vi "Construct.vi"(8 "error in":errorcluster, 11 "board properties in":T1 {"portConfig" items=["FDX_SINGLE", "FDX_REDUNDANT"]; "portSpeed" items=["FDX_100MBIT", "FDX_10MBIT", "FDX_AUTO_100MBIT", "FDX_AUTO_10MBIT", "FDX_AUTO_ERROR", "FDX_1000MBIT"]}) -> (0 "error out":errorcluster, 3 "Shared Resources out":refnum<class "Shared Resources.lvclass">)   [LabVIEW 2020, in "AIM ARINC 664 Engine.lvlib" / "Implementation.lvlib" / "Shared Resources.lvclass"]
uses:
  Shared Resources.lvclass
  Import/_typedefs/board_setup.ctl
  Import/AIM ARINC 664 Import.lvlib
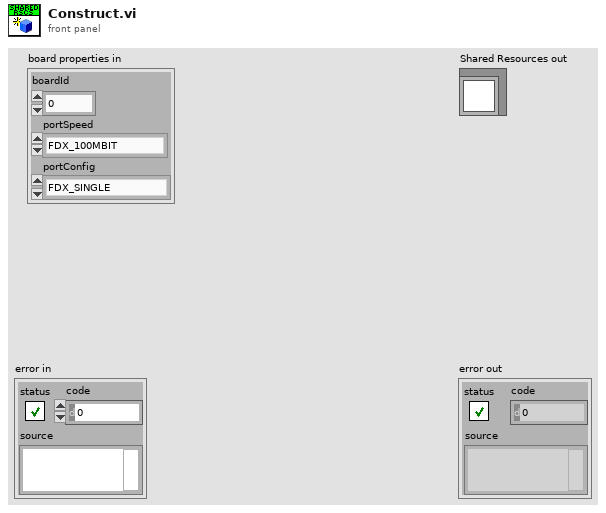
[diagram p1: front panel]
types:
  T1 = typedef "AIM ARINC 664 Import.lvlib/board_setup.ctl" = cluster{"boardId":u32, "portSpeed":u32, "portConfig":u32}
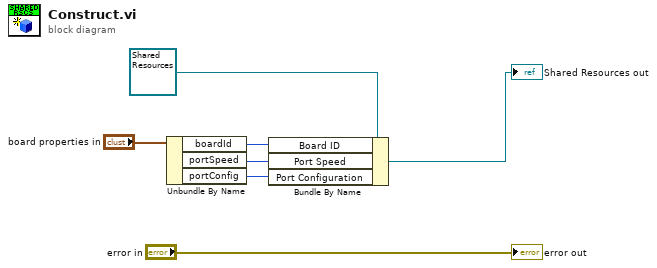
[diagram p0: block diagram]
diagram:
  n1 = Unbundle By Name("board properties in") -> ("boardId"=w3:u32, "portSpeed"=w2:u32, "portConfig"=w1:u32)
  n2 = Bundle By Name(cluster=refnum<class "Shared Resources.lvclass"> refnum ("Shared Resources in"), "Board ID"=w3, "Port Speed"=w2, "Port Configuration"=w1) -> (→"Shared Resources out":refnum<class "Shared Resources.lvclass">)
  "error out" <- "error in"
